vi "Volt Reader Trigger11.vi"() -> ()   [LabVIEW 2014]
uses:
  Enum State Machine Typedef.ctl
  <vilib>/Utility/error.llb/DialogType.ctl
  <vilib>/_DAQmxBase/Internals/DAQmxBase Create Channel (AI-Voltage-Basic).vi
  <vilib>/_DAQmxBase/Internals/DAQmxBase Timing (Sample Clock).vi
  <vilib>/measure/mamon.llb/Trigger Detection for 1 Channel.vi
  <vilib>/_DAQmxBase/Internals/DAQmxBase Read (Analog 2D DBL NChan NSamp).vi
  <vilib>/measure/NI_MAPro.lvlib
panel:
  out "Raw Graph":waveform(dbl)(graph)
  in  "Center":bool
  in  "Offset (percent of buffer)":dbl(knob) scale=-50.0..50.0
  in  "Timeout (in iterations)":i16
  out "State":T1
  out "Waveform Graph":waveform(dbl)(graph)
  in  "Buffer (Seconds)":dbl
  out "Threshold":dbl
  in  "units":i32(ring)=10348 items=["Volts"=10348, "From Custom Scale"=10065]
  in  "stop":bool
  in  "physical channels":tag
  in  "maximum value":dbl=5.0 format="%0.2f"
  in  "minimum value":dbl=-5.0 format="%0.2f"
  in  "rate":i32=1000 caption="Sample Rate"
  # "The inputs above MUST BE\nPreset before running"
  # "NOTE: Just change the Y axis value"
  # "Make Sure that Buffer does not equal 0"
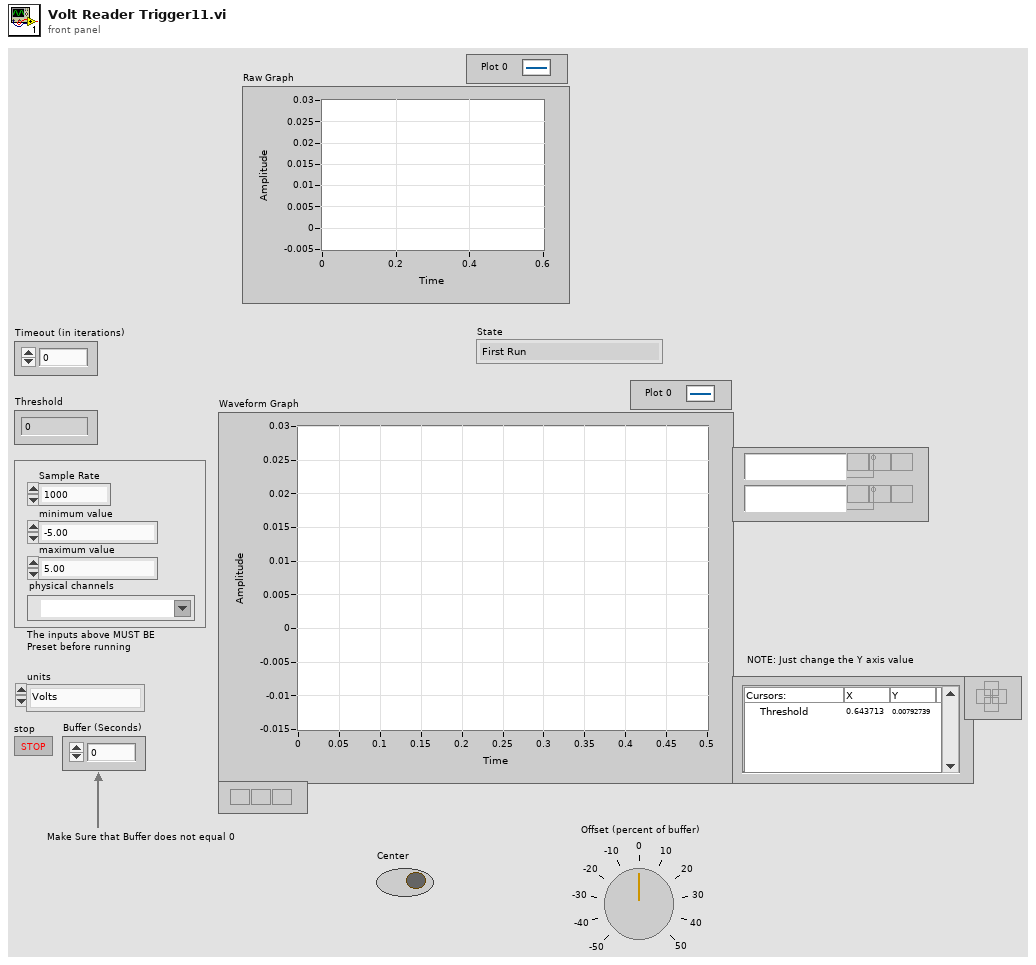
[diagram p1: front panel]
types:
  T1 = typedef "Enum State Machine Typedef.ctl" = enum16{"First Run", "Display Raw Data", "Gather and Edit Data", "Find Max with Gather Data", "Trigger Occured", "Found the Max", "Just Displayed", "The Max is in the Middle", "Base State", "Timeout"}
  T2 = typedef "DialogType.ctl" = u16
  T3 = typedef "LVCursorListTypeDef.ctl" = cluster{"Name":string, "Color":u32, "Style":u8, "Point Style":u8, "Name Visible":bool, "Allow Drag":bool, "Cursor Mode":u32, "Plot":i32, "Index":i32, "Position":cluster{"X":dbl, "Y":dbl}, "X Scale":u32, "Y Scale":u32, "Watch Plots":i32[], "Watch All Plots":bool, "Plot Area":i32, "Label Offset":cluster{"X":dbl, "Y":dbl}}[]
  T4 = cluster{"Name":string, "Color":u32, "Style":u8, "Point Style":u8, "Name Visible":bool, "Allow Drag":bool, "Cursor Mode":u32, "Plot":i32, "Index":i32, "Position":cluster{"X":dbl, "Y":dbl}, "X Scale":u32, "Y Scale":u32, "Watch Plots":i32[], "Watch All Plots":bool, "Plot Area":i32, "Label Offset":cluster{"X":dbl, "Y":dbl}}
  T5 = enum16{"In the Center Range", "Before the Center Range", "After the Center Range"}
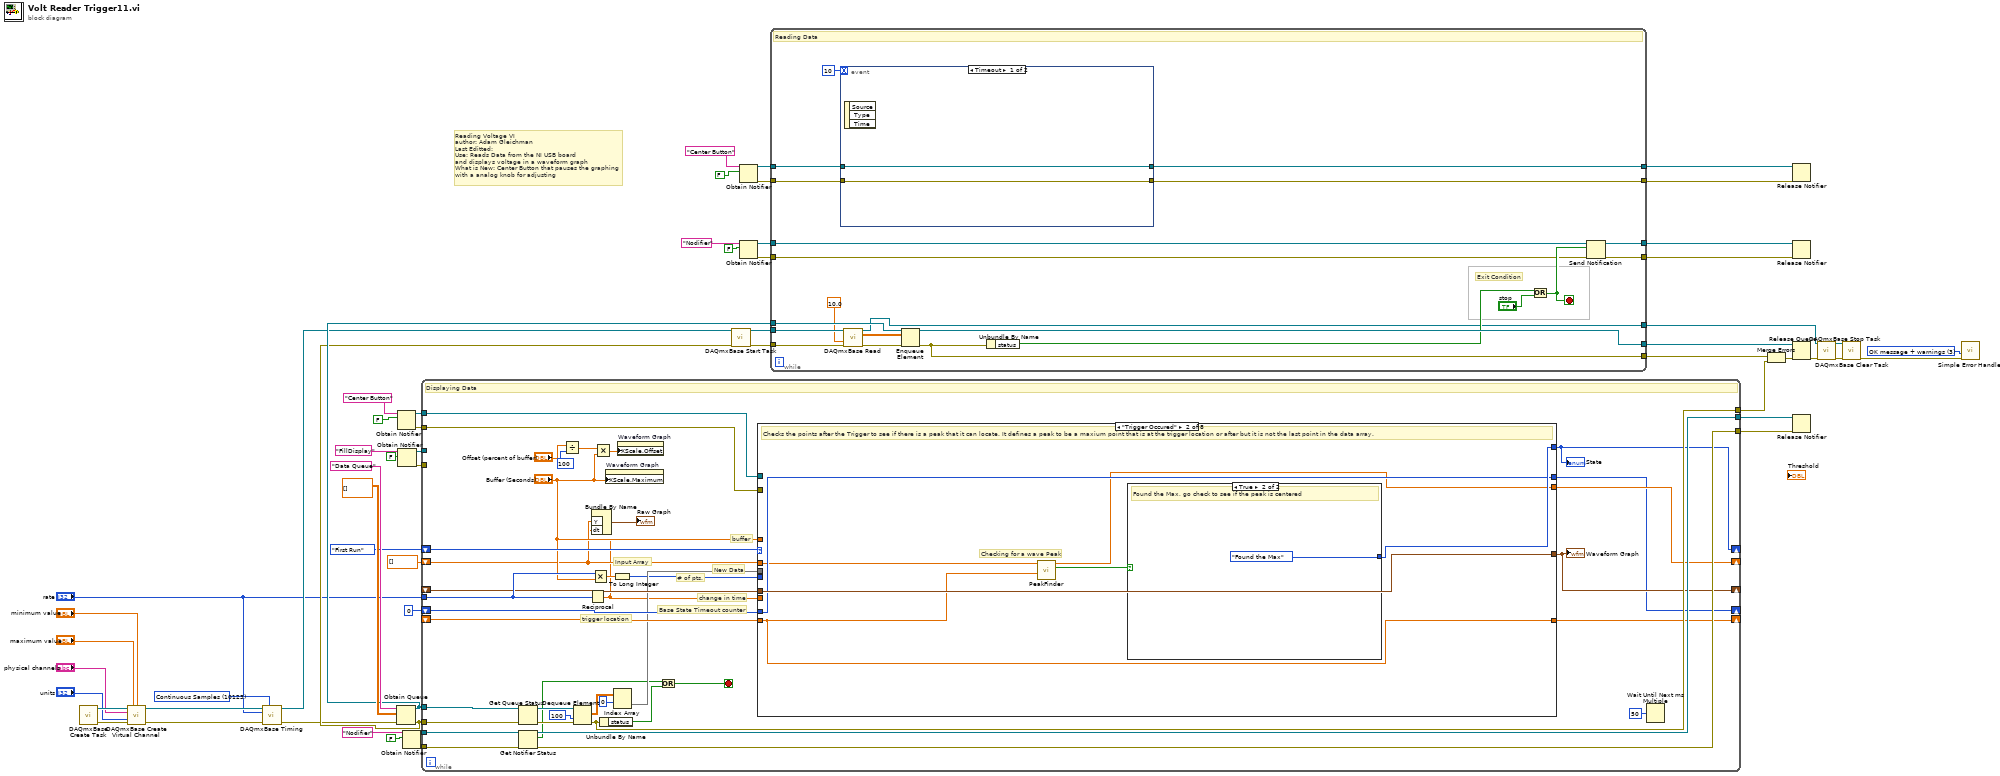
[diagram p0: block diagram]
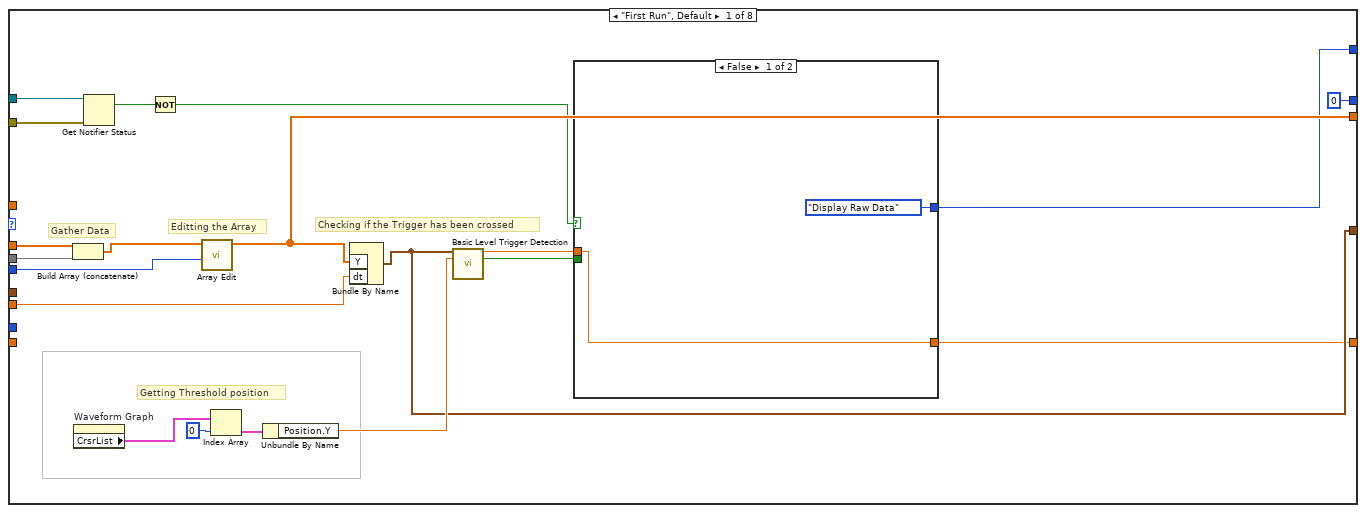
[diagram p2: hidden frame]
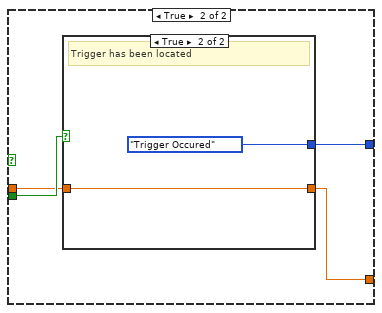
[diagram p3: hidden frame]
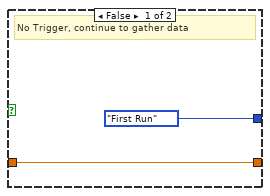
[diagram p4: hidden frame]
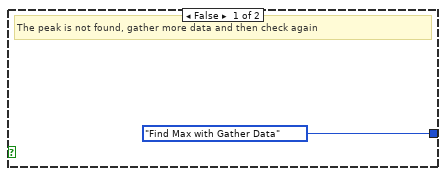
[diagram p5: hidden frame]
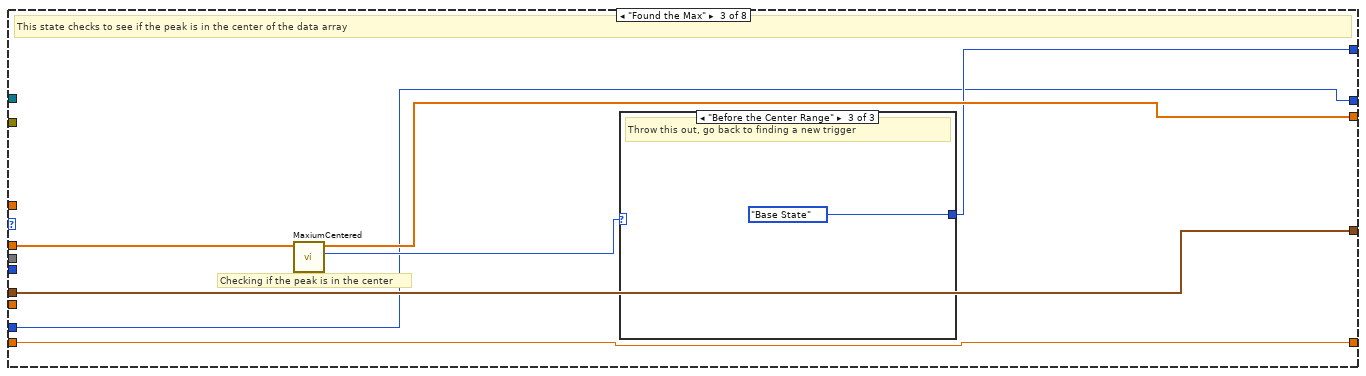
[diagram p6: hidden frame]
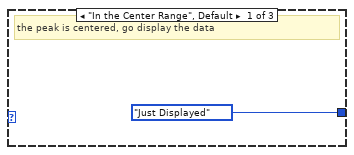
[diagram p7: hidden frame]
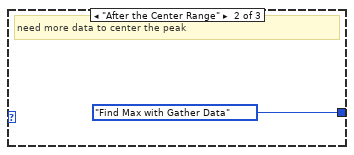
[diagram p8: hidden frame]
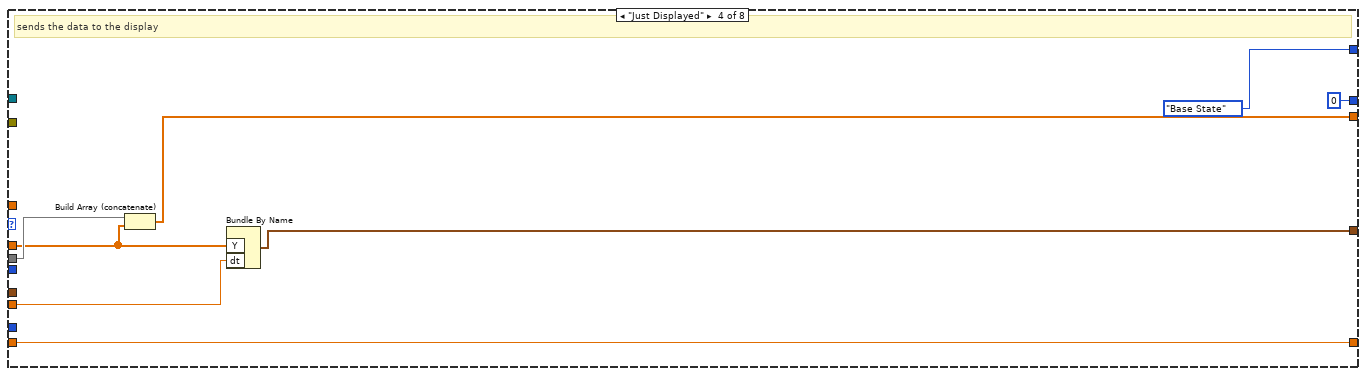
[diagram p9: hidden frame]
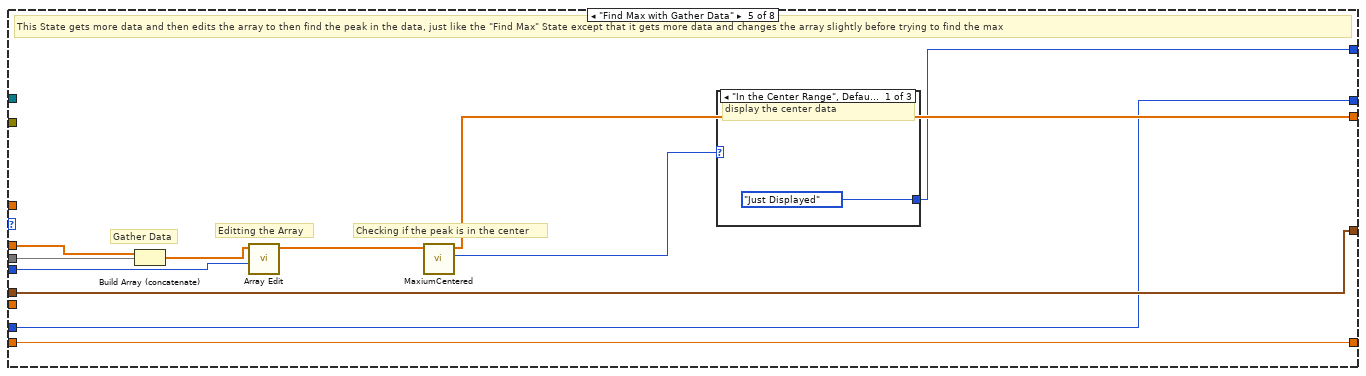
[diagram p10: hidden frame]
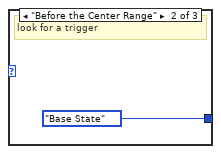
[diagram p11: hidden frame]
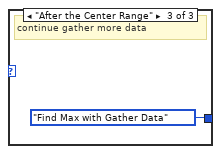
[diagram p12: hidden frame]
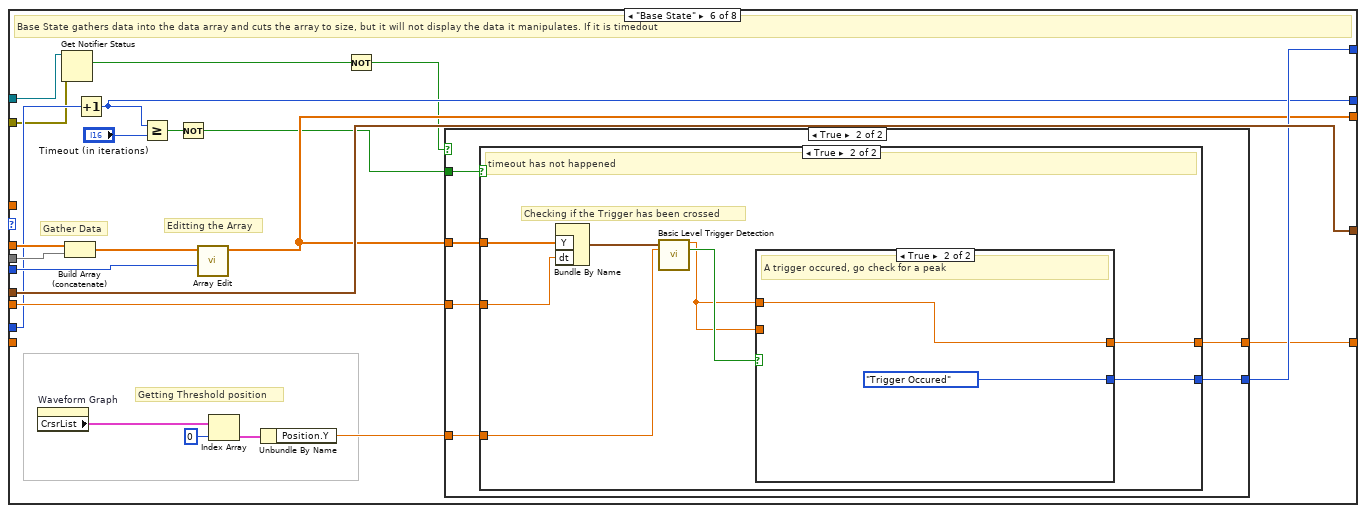
[diagram p13: hidden frame]
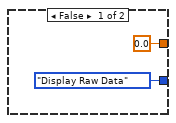
[diagram p14: hidden frame]
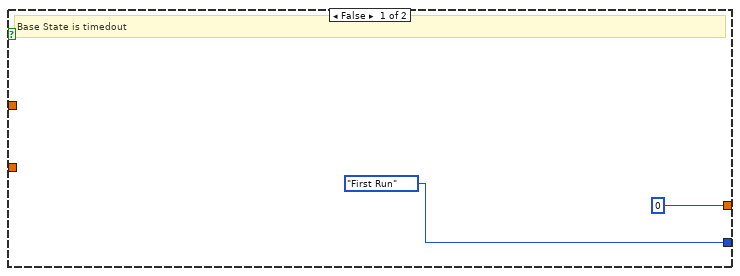
[diagram p15: hidden frame]
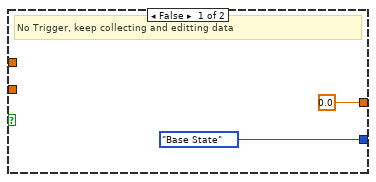
[diagram p16: hidden frame]
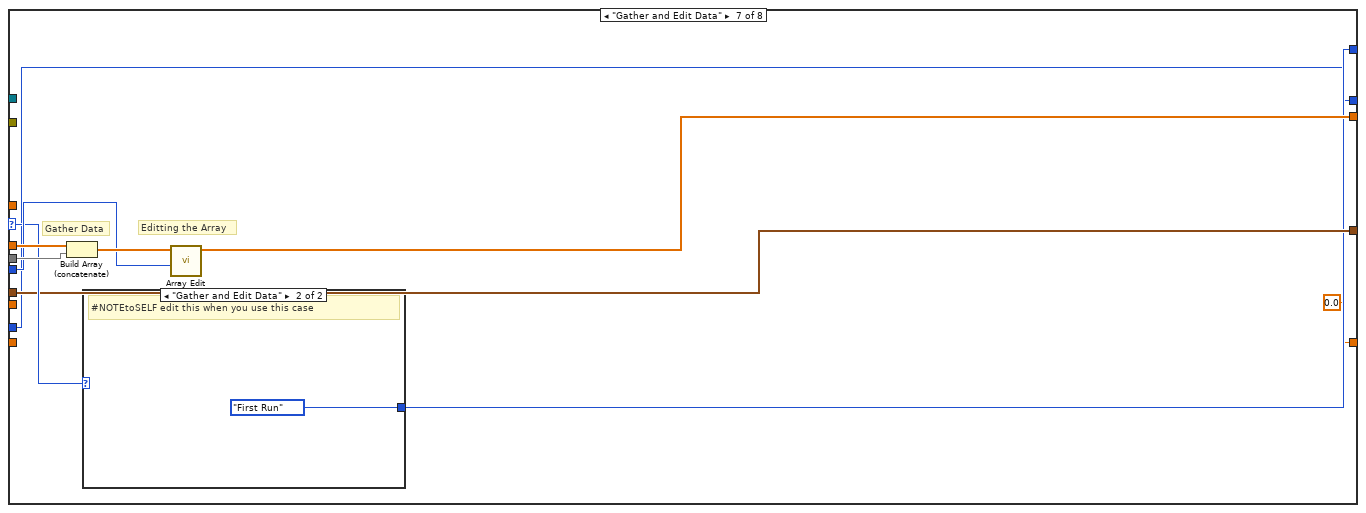
[diagram p17: hidden frame]
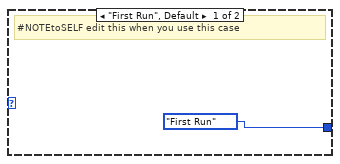
[diagram p18: hidden frame]
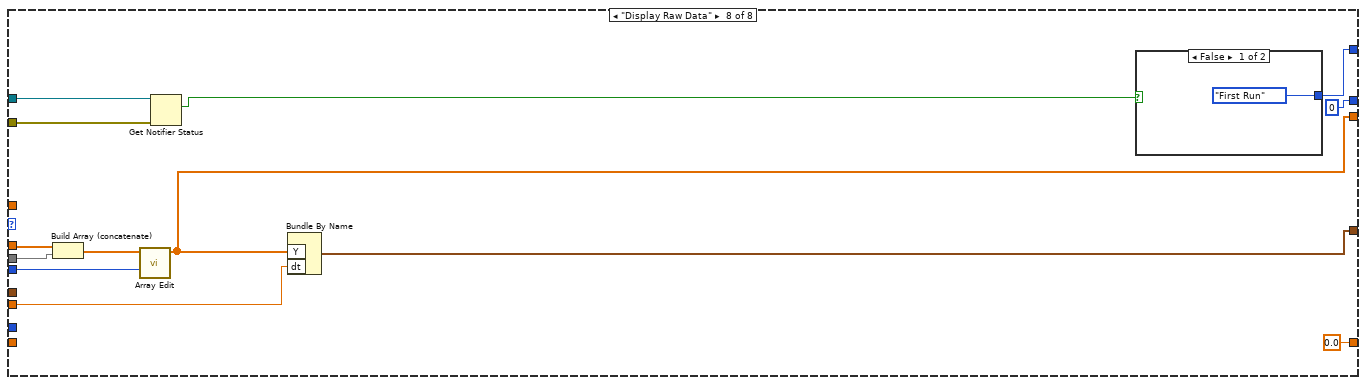
[diagram p19: hidden frame]
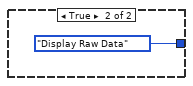
[diagram p20: hidden frame]
diagram:
  w34 = 10123 items=["Finite Samples"=10178, "Continuous Samples"=10123, "Hardware Timed Single Point"=12522] ("sample mode")
  w36 = T2 3 items=["no dialog", "OK message", "continue or stop message", "OK message + warnings", "continue/stop + warnings"] ("type of dialog (OK msg:1)")
  # "Reading Voltage VI\nauthor: Adam Gleichman\nLast Editted: \nUse: Reads Data from the NI USB board\nand displays voltage in a waveform graph\nWhat is New: Center Button that pauses the graphing\nwith a analog knob for adjusting"
  n1 = call <vilib>:"DAQmxBase Create Task.vi"() -> ("task out"=w56:refnum<k21>, "error out"=w55:errorcluster)  [unwired: 5 in, 9 out]
  n2 = call-poly <vilib>:"DAQmxBase Create Virtual Channel.vi"("task in"=w56, "maximum value"="maximum value", "minimum value"="minimum value", "physical channels"="physical channels", "units"="units", "error in"=w55) -> ("task out"=w53:refnum<k21>, "error out"=w54:errorcluster)  [unwired: 3 in, 5 out]
  n3 = call-poly <vilib>:"DAQmxBase Timing.vi"("task/channels in"=w53, "sample mode"=w34, "rate"="rate", "error in"=w54) -> ("task out"=w22:refnum<k21>, "error out"=w21:errorcluster)  [unwired: 3 in, 7 out]
  n4 = Obtain Queue(name (unnamed)="Data Queue", element data type=dbl[][] [] ("data"), error in (no error)=w21) -> (queue out=w43:refnum<queue>, error out=w42:errorcluster)  [unwired: 2 in, 1 out]
  n5 = Obtain Notifier(name (unnamed)="Center Button", notification data type=FALSE) -> (notifier out=w4:refnum<notifier>, error out=w3:errorcluster)  [unwired: 2 in, 1 out]
  n6 = Obtain Notifier(name (unnamed)="FillDisplay", notification data type=FALSE) -> (notifier out=w18:refnum<notifier>, error out=w17:errorcluster)  [unwired: 2 in, 1 out]
  n7 = Obtain Notifier(name (unnamed)="Nodifier", notification data type=FALSE) -> (notifier out=w27:refnum<notifier>, error out=w25:errorcluster)  [unwired: 2 in, 1 out]
  n8 = while {
    tunnel: w43 -> [w96]
    tunnel: w42 -> [w87]
    tunnel: [w94] -> w41
    tunnel: w27 -> [w92]
    tunnel: w25 -> [w91]
    tunnel: [w90] -> w23
    tunnel: [w89] -> w24
    tunnel: "rate" -> [w83]
    shift-right: [w78] -> _
    shift-left: dbl[] [] -> [w60]
    tunnel: w18 -> [_]
    tunnel: w17 -> [_]
    shift-right: [w77] -> _
    shift-left: Enum_State_Machine_Typedef."First Run" -> [w80]
    shift-right: [w79] -> _
    shift-left: _ -> [w81]
    shift-right: [w75] -> _
    shift-left: 0 -> [w76]
    shift-right: [w74] -> _
    shift-left: _ -> [w73]
    tunnel: w4 -> [w63]
    tunnel: w3 -> [w62]
    stop <- w93 stop-if-true
    # "trigger location"
    # "change in time"
    # "buffer"
    # "Base State Timeout counter"
    # "New Data"
    # "Input Array"
    # "# of pts."
    # "Displaying Data"
    n9 = Get Queue Status(queue=w96, error in (no error)=w87) -> (queue out=w88:refnum<queue>, error out=w86:errorcluster)  [unwired: 1 in, 6 out]
    n10 = Get Notifier Status(notifier=w92, error in (no error)=w91) -> (notifier out=w90:refnum<notifier>, current notification=w64:bool, error out=w89:errorcluster)  [unwired: 2 out]
    n11 = Divide(x="Offset (percent of buffer)", y=100) -> (x/y=w67:dbl)
    n12 = Dequeue Element(queue=w88, timeout in ms (-1)=100, error in (no error)=w86) -> (element=w84:dbl[][], error out=w94:errorcluster)  [unwired: 2 out]
    n13 = Reciprocal(x=w83) -> (1/x=w59:dbl)
    n14 = Bundle By Name("Y"=w60, "dt"=w59) -> (→"Raw Graph":waveform(dbl))  [unwired: 1 in]
    n15 = Multiply(x=w83, y="Buffer (Seconds)") -> (x*y=w82:dbl)
    n16 = Multiply(x=w67, y="Buffer (Seconds)") -> (x*y=w66:dbl)
    n17 = Unbundle By Name(w94) -> ("status"=w65:bool)
    n18 = property on="Waveform Graph" class="WFGraph (strict)"("XScale.Maximum"="Buffer (Seconds)") -> ()  [unwired: 2 in, 2 out]
    n19 = To Long Integer(number=w82) -> (32bit integer=w71:i32)
    n20 = Index Array(array=w84, index (row)=0 ("index")) -> (element=w72:dbl[])  [unwired: 1 in]
    n21 = property on="Waveform Graph" class="WFGraph (strict)"("XScale.Offset"=w66) -> ()  [unwired: 2 in, 2 out]
    n22 = Or(x=w64, y=w65) -> (x .or. y?=w93:bool)
    n23 = case shown="\"Trigger Occured\"" w80 {
      selector: w80 -> [_ _ _ _ _ _ w217 _]
      tunnel: w60 -> [w116 w130 w142 w146 w164 w189 w221 w236]
      tunnel: w72 -> [w115 _ _ w147 w163 w188 w220 w235]
      tunnel: w59 -> [w109 _ _ w153 _ w182 _ w232]
      tunnel: w71 -> [w113 _ _ _ w161 w186 w218 w233]
      tunnel: [w106 w133 w138 w151 w156 w181 w215 w225] -> w79
      tunnel: w81 -> [_ w133 w138 _ w156 w181 w215 _]
      tunnel: "Buffer (Seconds)" -> [_ _ _ _ _ _ _ _]
      tunnel: [w105 w129 w141 w152 w158 w179 w216 w224] -> w78
      tunnel: [w104 w132 w139 Enum_State_Machine_Typedef."Base State" w157 w180 w214 w228] -> w77
      tunnel: w76 -> [_ w131 w136 _ w155 w177 w213 _]
      tunnel: [0 w131 w136 0 w155 w173 w213 0] -> w75
      tunnel: [w102 w127 w137 w149 w154 w172 0.0 ("trigger location") 0.0 ("trigger location")] -> w74
      tunnel: w73 -> [_ w127 w137 w149 w154 _ _ _]
      tunnel: w63 -> [w100 _ _ _ _ w171 _ w231]
      tunnel: w62 -> [w99 _ _ _ _ w170 _ w230]
      frame "First Run", Default {
        # "Checking if the Trigger has been crossed"
        # "Getting Threshold position"
        # "Editting the Array"
        # "Gather Data"
        n24 = Build Array (concatenate)(w116, w115) -> (w114:dbl[])
        n25 = property on="Waveform Graph" class="WFGraph (strict)"() -> ("CrsrList"=w111:T3)  [unwired: 2 in, 2 out]
        n26 = Get Notifier Status(notifier=w100, error in (no error)=w99) -> (current notification=w98:bool)  [unwired: 4 out]
        n27 = Not(x=w98) -> (.not. x?=w97:bool)
        n28 = call "Array Edit.vi"("Number of Points"=w113, "Y-values"=w114) -> ("Editted Y Values"=w105:dbl[])  [unwired: 9 in]
        n29 = Index Array(array=w111, index=0) -> (element=w112:T4)
        n30 = Unbundle By Name(w112) -> ("Position.Y"=w108:dbl)
        n31 = Bundle By Name("Y"=w105, "dt"=w109) -> (w106:waveform(dbl))  [unwired: 1 in]
        n32 = call-poly <vilib>:"Basic Level Trigger Detection.vi"("signal in"=w106, "level"=w108) -> ("trigger location"=w103:dbl, "trigger detected?"=w107:bool)  [unwired: 11 in, 1 out]
        n33 = case shown="False" w97 {
          tunnel: w107 -> [_ w122]
          tunnel: [Enum_State_Machine_Typedef."Display Raw Data" w121] -> w104
          tunnel: w103 -> [w118 w120]
          tunnel: [w118 w119] -> w102
          frame False {
          }
          frame True {
            n34 = case shown="True" w122 {
              tunnel: [Enum_State_Machine_Typedef."First Run" Enum_State_Machine_Typedef."Trigger Occured"] -> w121
              tunnel: w120 -> [w123 w125]
              tunnel: [w123 w125] -> w119
              frame False {
                # "No Trigger, continue to gather data"
              }
              frame True {
                # "Trigger has been located"
              }
            }
          }
        }
      }
      frame "Trigger Occured" {
        # "Checking for a wave Peak"
        # "Checks the points after the Trigger to see if there is a peak that it can locate. It defines a peak to be a maxium point that is at the trigger location or after but it is not the last point in the data array."
        n35 = call "PeakFinder.vi"("Trigger location"=w127, "Input Y values"=w130) -> ("peak?"=w128:bool, "Input Y values"=w129:dbl[])  [unwired: 8 in]
        n36 = case shown="True" w128 {
          tunnel: [Enum_State_Machine_Typedef."Find Max with Gather Data" Enum_State_Machine_Typedef."Found the Max"] -> w132
          frame False {
            # "The peak is not found, gather more data and then check again"
          }
          frame True {
            # "Found the Max, go check to see if the peak is centered"
          }
        }
      }
      frame "Found the Max" {
        # "Checking if the peak is in the center"
        # "This state checks to see if the peak is in the center of the data array"
        n37 = call "MaxiumCentered.vi"("Input Y Values"=w142) -> ("State output"=w140:T5, "Output Y Values"=w141:dbl[])  [unwired: 9 in]
        n38 = case shown="\"Before the Center Range\"" w140 {
          tunnel: [Enum_State_Machine_Typedef."Just Displayed" Enum_State_Machine_Typedef."Find Max with Gather Data" Enum_State_Machine_Typedef."Base State"] -> w139
          frame "In the Center Range", Default {
            # "the peak is centered, go display the data"
          }
          frame "After the Center Range" {
            # "need more data to center the peak"
          }
          frame "Before the Center Range" {
            # "Throw this out, go back to finding a new trigger"
          }
        }
      }
      frame "Just Displayed" {
        # "sends the data to the display"
        n39 = Build Array (concatenate)(w147, w146) -> (w152:dbl[])
        n40 = Bundle By Name("Y"=w146, "dt"=w153) -> (w151:waveform(dbl))  [unwired: 1 in]
      }
      frame "Find Max with Gather Data" {
        # "Editting the Array"
        # "Gather Data"
        # "Checking if the peak is in the center"
        # "This State gets more data and then edits the array to then find the peak in the data, just like the \"Find Max\" State except that it gets more data and changes the array slightly before trying to find the max"
        n41 = Build Array (concatenate)(w164, w163) -> (w162:dbl[])
        n42 = call "Array Edit.vi"("Number of Points"=w161, "Y-values"=w162) -> ("Editted Y Values"=w160:dbl[])  [unwired: 9 in]
        n43 = call "MaxiumCentered.vi"("Input Y Values"=w160) -> ("State output"=w159:T5, "Output Y Values"=w158:dbl[])  [unwired: 9 in]
        n44 = case shown="\"In the Center Range\", Default" w159 {
          tunnel: [Enum_State_Machine_Typedef."Just Displayed" Enum_State_Machine_Typedef."Base State" Enum_State_Machine_Typedef."Find Max with Gather Data"] -> w157
          frame "In the Center Range", Default {
            # "display the center data"
          }
          frame "Before the Center Range" {
            # "look for a trigger"
          }
          frame "After the Center Range" {
            # "continue gather more data"
          }
        }
      }
      frame "Base State" {
        # "Getting Threshold position"
        # "Editting the Array"
        # "Gather Data"
        # "Base State gathers data into the data array and cuts the array to size, but it will not display the data it manipulates. If it is timedout"
        n45 = property on="Waveform Graph" class="WFGraph (strict)"() -> ("CrsrList"=w178:T3)  [unwired: 2 in, 2 out]
        n46 = Get Notifier Status(notifier=w171, error in (no error)=w170) -> (current notification=w169:bool)  [unwired: 4 out]
        n47 = Build Array (concatenate)(w189, w188) -> (w187:dbl[])
        n48 = Increment(x=w177) -> (x+1=w173:i32)
        n49 = Greater Or Equal?(x=w173, y="Timeout (in iterations)") -> (x >= y?=w175:bool)
        n50 = Not(x=w175) -> (.not. x?=w174:bool)
        n51 = call "Array Edit.vi"("Number of Points"=w186, "Y-values"=w187) -> ("Editted Y Values"=w179:dbl[])  [unwired: 9 in]
        n52 = Index Array(array=w178, index=0) -> (element=w185:T4)
        n53 = Unbundle By Name(w185) -> ("Position.Y"=w183:dbl)
        n54 = Not(x=w169) -> (.not. x?=w168:bool)
        n55 = case shown="True" w168 {
          tunnel: w183 -> [_ w197]
          tunnel: w182 -> [_ w196]
          tunnel: [Enum_State_Machine_Typedef."Display Raw Data" w195] -> w180
          tunnel: w179 -> [_ w194]
          tunnel: w174 -> [_ w193]
          tunnel: [0.0 ("trigger location") w192] -> w172
          frame False {
          }
          frame True {
            n56 = case shown="True" w193 {
              tunnel: w197 -> [_ w206]
              tunnel: w196 -> [_ w205]
              tunnel: [Enum_State_Machine_Typedef."First Run" w203] -> w195
              tunnel: w194 -> [_ w202]
              tunnel: [0 w200] -> w192
              frame False {
                # "Base State is timedout"
              }
              frame True {
                # "Checking if the Trigger has been crossed"
                # "timeout has not happened"
                n57 = Bundle By Name("Y"=w202, "dt"=w205) -> (w207:waveform(dbl))  [unwired: 1 in]
                n58 = call-poly <vilib>:"Basic Level Trigger Detection.vi"("signal in"=w207, "level"=w206) -> ("trigger location"=w201:dbl, "trigger detected?"=w204:bool)  [unwired: 11 in, 1 out]
                n59 = case shown="True" w204 {
                  tunnel: [Enum_State_Machine_Typedef."Base State" Enum_State_Machine_Typedef."Trigger Occured"] -> w203
                  tunnel: w201 -> [_ _]
                  tunnel: [0.0 w210] -> w200
                  tunnel: w201 -> [_ w210]
                  frame False {
                    # "No Trigger, keep collecting and editting data"
                  }
                  frame True {
                    # "A trigger occured, go check for a peak"
                  }
                }
              }
            }
          }
        }
      }
      frame "Gather and Edit Data" {
        # "Editting the Array"
        # "Gather Data"
        n60 = Build Array (concatenate)(w221, w220) -> (w219:dbl[])
        n61 = case shown="\"Gather and Edit Data\"" w217 {
          tunnel: [Enum_State_Machine_Typedef."First Run" Enum_State_Machine_Typedef."First Run"] -> w214
          frame "First Run", Default {
            # "#NOTEtoSELF edit this when you use this case"
          }
          frame "Gather and Edit Data" {
            # "#NOTEtoSELF edit this when you use this case"
          }
        }
        n62 = call "Array Edit.vi"("Number of Points"=w218, "Y-values"=w219) -> ("Editted Y Values"=w216:dbl[])  [unwired: 9 in]
      }
      frame "Display Raw Data" {
        n63 = Build Array (concatenate)(w236, w235) -> (w234:dbl[])
        n64 = call "Array Edit.vi"("Number of Points"=w233, "Y-values"=w234) -> ("Editted Y Values"=w224:dbl[])  [unwired: 9 in]
        n65 = Get Notifier Status(notifier=w231, error in (no error)=w230) -> (current notification=w229:bool)  [unwired: 4 out]
        n66 = Bundle By Name("Y"=w224, "dt"=w232) -> (w225:waveform(dbl))  [unwired: 1 in]
        n67 = case shown="False" w229 {
          tunnel: [Enum_State_Machine_Typedef."First Run" Enum_State_Machine_Typedef."Display Raw Data"] -> w228
          frame False {
          }
          frame True {
          }
        }
      }
    }
    "Waveform Graph" <- w79
    "State" <- w77
    n68 = Wait Until Next ms Multiple(millisecond multiple=u32 50) -> ()  [unwired: 1 out]
  }
  n69 = call <vilib>:"DAQmxBase Start Task.vi"("task/channels in"=w22, "error in"=w42) -> ("task out"=w51:refnum<k21>, "error out"=w52:errorcluster)  [unwired: 12 out]
  n70 = Obtain Notifier(name (unnamed)="Center Button", notification data type=FALSE) -> (notifier out=w10:refnum<notifier>, error out=w9:errorcluster)  [unwired: 2 in, 1 out]
  n71 = Obtain Notifier(name (unnamed)="Nodifier", notification data type=FALSE) -> (notifier out=w30:refnum<notifier>, error out=w29:errorcluster)  [unwired: 2 in, 1 out]
  n72 = while "Data Reading Loop" {
    tunnel: w52 -> [w258]
    tunnel: w51 -> [w259]
    tunnel: w43 -> [w256]
    tunnel: [w253] -> w46
    tunnel: [w251] -> w45
    tunnel: [w249] -> w33
    tunnel: w30 -> [w247]
    tunnel: w29 -> [w246]
    tunnel: [w245] -> w20
    tunnel: [w244] -> w19
    tunnel: w10 -> [w243]
    tunnel: w9 -> [w242]
    tunnel: [w241] -> w2
    tunnel: [w240] -> w1
    stop <- w248 stop-if-true
    # "Exit Condition"
    # "Reading Data"
    n73 = event shown="[0] Timeout" {
      selector: _ -> [_ _]
      dyn-events: _ -> [_ _]
      timeout: 10 -> [_ _]
      tunnel: w243 -> [w261 w266]
      tunnel: w242 -> [w260 w265]
      tunnel: [w261 w263] -> w241
      tunnel: [w260 w262] -> w240
      event Timeout {
        n74 = event-data() -> ()  [unwired: 1 in, 3 out]
      }
      event "Center": Value Change {
        n75 = event-data() -> ()  [unwired: 1 in, 1 out]
        n76 = Send Notification(notification="Center", notifier=w266, error in (no error)=w265) -> (notifier out=w263:refnum<notifier>, error out=w262:errorcluster)
      }
    }
    n77 = call-poly <vilib>:"DAQmxBase Read.vi"("task/channels in"=w259, "timeout"=10.0, "error in"=w258) -> ("task out"=w249:refnum<k21>, "data"=w254:dbl[][], "error out"=w257:errorcluster)  [unwired: 10 in]
    n78 = Enqueue Element(queue=w256, element=w254, error in (no error)=w257) -> (queue out=w253:refnum<queue>, error out=w251:errorcluster)  [unwired: 1 in, 1 out]
    n79 = Unbundle By Name(w251) -> ("status"=w250:bool)
    n80 = Or(x=w250, y="stop") -> (x .or. y?=w248:bool)
    n81 = Send Notification(notification=w248, notifier=w247, error in (no error)=w246) -> (notifier out=w245:refnum<notifier>, error out=w244:errorcluster)
  }
  n82 = Merge Errors(w45, w41) -> (w44:errorcluster)
  n83 = Release Notifier(notifier=w2, error in (no error)=w1) -> ()  [unwired: 1 in, 3 out]
  n84 = Release Notifier(notifier=w20, error in (no error)=w19) -> ()  [unwired: 1 in, 3 out]
  n85 = Release Queue(queue=w46, error in (no error)=w44) -> (error out=w40:errorcluster)  [unwired: 1 in, 2 out]
  n86 = Release Notifier(notifier=w23, error in (no error)=w24) -> ()  [unwired: 1 in, 3 out]
  n87 = call <vilib>:"DAQmxBase Stop Task.vi"("task/channels in"=w33, "error in"=w40) -> ("task out"=w39:refnum<k21>, "error out"=w38:errorcluster)  [unwired: 12 in]
  n88 = call <vilib>:"DAQmxBase Clear Task.vi"("task in"=w39, "error in"=w38) -> ("error out"=w37:errorcluster)  [unwired: 13 in]
  n89 = call <vilib>:"Simple Error Handler.vi"("type of dialog (OK msg:1)"=w36, "error in (no error)"=w37) -> ()  [unwired: 3 in, 5 out]
